vi "Cycling status.vi"(8 "error in":errorcluster, 9 "Enum":T1, 10 "Triggered?":bool, 11 "RPM":dbl) -> (0 "error out":errorcluster)   [LabVIEW 2020, in "Cycling by State module.lvlib"]
doc: "Update cycling status\n_____\nCreated using DQMH Event Scripter 7.0.1.1316."
uses:
  Cycling by State module.lvlib
  Cycling state.ctl
  Cycling status Argument--cluster.ctl
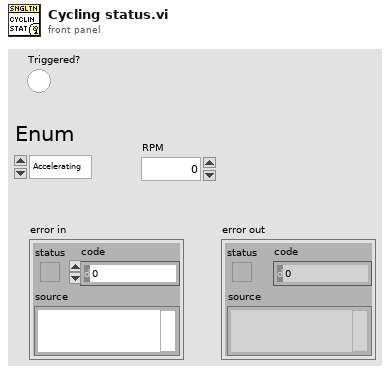
[diagram p1: front panel]
types:
  T1 = typedef "Cycling by State module.lvlib/Cycling state.ctl" = enum16{"Accelerating", "Detecting 100rpm", "Pressing until 0rpm"}
  T2 = typedef "Cycling by State module.lvlib/Cycling status Argument--cluster.ctl" = cluster{"Triggered?":bool, "Enum":T1, "RPM":dbl}
  T3 = typedef "Cycling by State module.lvlib/Broadcast Events--cluster.ctl" = cluster{"Module Did Init":refnum<user-event>, "Status Updated":refnum<user-event>, "Error Reported":refnum<user-event>, "Module Did Stop":refnum<user-event>, "Update Module Execution Status":refnum<user-event>, "Cycling status":refnum<user-event>}
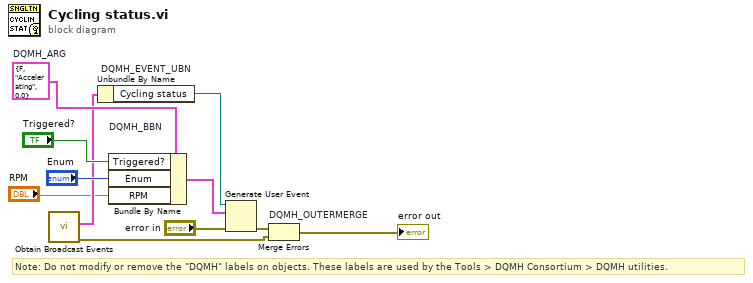
[diagram p0: block diagram]
diagram:
  w6 = T2 {"Triggered?"=FALSE, "Enum"=enum."Accelerating", "RPM"=0.0}  # DQMH_ARG
  # "Note: Do not modify or remove the \"DQMH\" labels on objects. These labels are used by the Tools > DQMH Consortium > DQMH utilities."
  n1 = call "Obtain Broadcast Events.vi"() -> ("error out"=w3:errorcluster, "Cycling by State module Broadcast Events"=w2:T3)  [unwired: 10 in]
  n2 = Unbundle By Name "DQMH_EVENT_UBN"(w2) -> ("Cycling status"=w8:refnum<user-event>)
  n3 = Bundle By Name "DQMH_BBN"(cluster=w6, "Triggered?"="Triggered?", "Enum"="Enum", "RPM"="RPM") -> (w9:T2)
  n4 = Generate User Event(user event=w8, event data cluster=w9, error in="error in") -> (error out=w7:errorcluster)  [unwired: 1 in, 1 out]
  n5 = Merge Errors "DQMH_OUTERMERGE"(w7, w3) -> (→"error out":errorcluster)
